vi "Get All Nodes.vi"(8 "error in (no error)":errorcluster, 11 "List in":refnum<class "DoubleLinkedList.lvclass">) -> (0 "error out":errorcluster, 2 "Array":refnum<class "ListNode.lvclass">[](array[class]), 3 "List out":refnum<class "DoubleLinkedList.lvclass">)   [LabVIEW 2010, in "DoubleLinkedList.lvclass"]
uses:
  DoubleLinkedList.lvclass
  ListNode/ListNode.lvclass
  DoubleLinkedList.lvclass/DoubleLinkedList.ctl
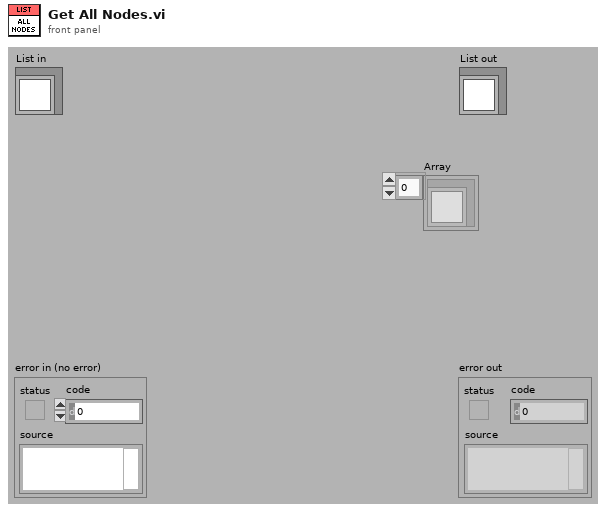
[diagram p1: front panel]
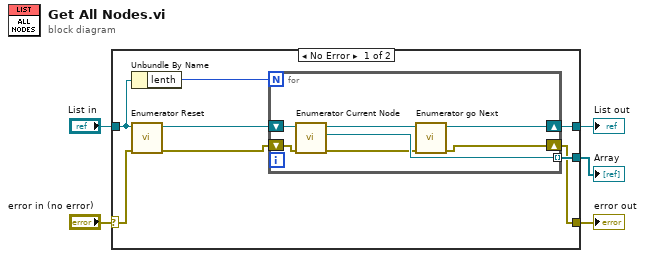
[diagram p0: block diagram]
diagram:
  n1 = case shown="No Error" "error in (no error)" {
    selector: "error in (no error)" -> [w9 w22]
    tunnel: [w7 w22] -> w4
    tunnel: [w11 w21] -> w2
    tunnel: "List in" -> [w13 w21]
    tunnel: [w10 _] -> w1
    frame No Error {
      n2 = Unbundle By Name(w13) -> ("lenth"=w6:u32)
      n3 = call-dynamic "Enumerator Reset.vi"("error in (no error)"=w9, "List in"=w13) -> ("error out"=w8:errorcluster, "List out"=w12:refnum<class "DoubleLinkedList.lvclass">)  [unwired: 8 in]
      n4 = for {
        N: w6 -> [_]
        shift-right: [w17] -> w11
        shift-left: w12 -> [w19]
        tunnel: [w20] -> w10 mode=indexing
        shift-right: [w14] -> w7
        shift-left: w8 -> [w16]
        n5 = call-dynamic "Enumerator Current Node.vi"("error in (no error)"=w16, "List in"=w19) -> ("error out"=w15:errorcluster, "Node"=w20:refnum<class "ListNode.lvclass">, "List out"=w18:refnum<class "DoubleLinkedList.lvclass">)  [unwired: 7 in]
        n6 = call-dynamic "Enumerator go Next.vi"("error in (no error)"=w15, "List in"=w18) -> ("error out"=w14:errorcluster, "List out"=w17:refnum<class "DoubleLinkedList.lvclass">)  [unwired: 8 in]
      }
    }
    frame Error {
    }
  }
  "error out" <- w4
  "List out" <- w2
  "Array" <- w1
